vi "form_template.vi"(11 "JSON":string) -> ()   [LabVIEW 2021]
doc: "Form template VI.\n\nWhen you want to create a new form, please copy and modify this VI.\nThe form vi should be placed in the host/form directory."
uses:
  host/core/host_global_vars.vi
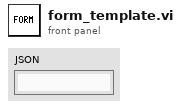
[diagram p1: front panel]
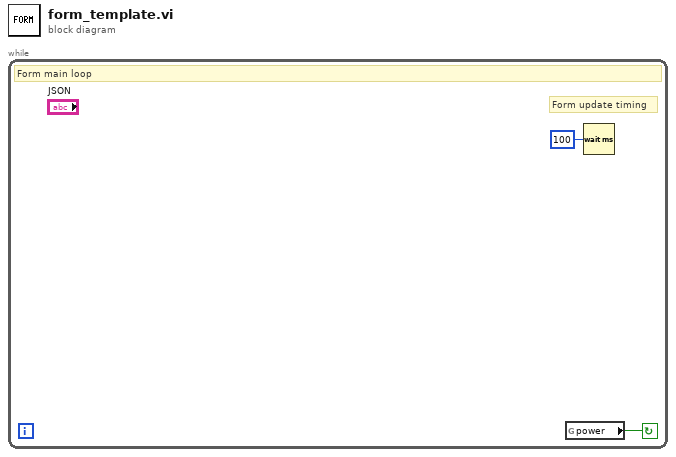
[diagram p0: block diagram]
diagram:
  n1 = while {
    stop <- w2 continue-if-true
    # "Form update timing"
    # "Form main loop"
    n2 = global read "host_global_vars.vi" "power"() -> (w2:bool)
    n3 = Wait (ms)(milliseconds to wait=u32 100) -> ()  [unwired: 1 out]
  }
